vi "dvr_fgv.vi"(8 "error in (no error)":errorcluster) -> (0 "error out":errorcluster, 3 "data value reference":refnum<data-value>)   [LabVIEW 2020]
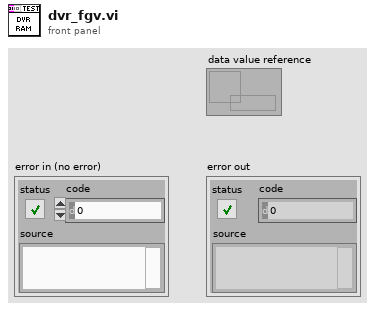
[diagram p1: front panel]
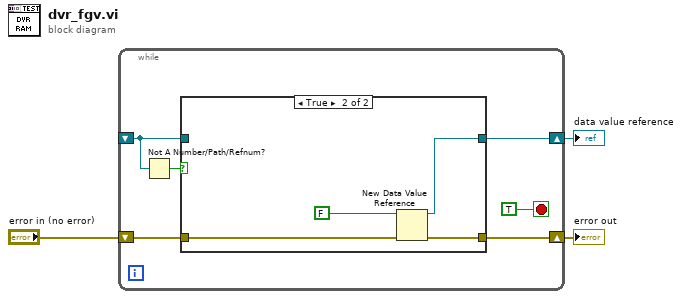
[diagram p0: block diagram]
diagram:
  n1 = while {
    shift-right: [w7] -> w2
    shift-left: "error in (no error)" -> [w8]
    shift-right: [w6] -> w1
    shift-left: _ -> [w4]
    stop <- TRUE stop-if-true
    n2 = Not A Number/Path/Refnum?(number/path/refnum=w4) -> (NaN/Path/Refnum?=w5:bool)
    n3 = case shown="True" w5 {
      tunnel: w8 -> [w10 w15]
      tunnel: [w10 w14] -> w7
      tunnel: [w11 w13] -> w6
      tunnel: w4 -> [w11 _]
      frame False {
      }
      frame True {
        n4 = New Data Value Reference(data value=FALSE, error in=w15) -> (data value reference=w13:refnum<data-value>, error out=w14:errorcluster)
      }
    }
  }
  "error out" <- w2
  "data value reference" <- w1
